vi "打开关闭文件_夹.vi"(8 "仅选中":bool, 9 "路径":path=path "C:/Users/Administrator/Desktop/技术资料/上位机/烧写软件/WR901_UpgradeTools_V3.1.3_User_20171115发布/UpgradeTools.exe", 10 "打开/关闭T":bool=TRUE, 11 "wait until completion? (T)":bool caption="等待结果后结束？(F)") -> ()   [LabVIEW 2015]
panel:
  out "standard output":string caption="标准输出"
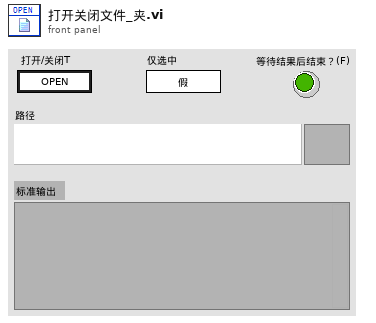
[diagram p1: front panel]
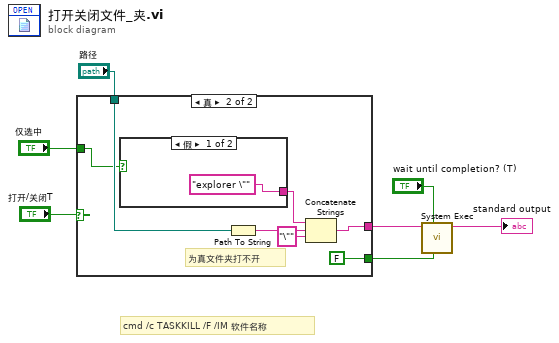
[diagram p0: block diagram]
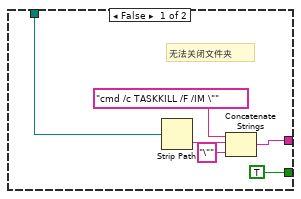
[diagram p2: hidden frame]
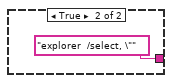
[diagram p3: hidden frame]
diagram:
  # "cmd /c TASKKILL /F /IM 软件名称"
  n1 = case shown="真" "打开/关闭T" {
    tunnel: [w12 w17] -> w7
    tunnel: "路径" -> [w11 w19]
    tunnel: [TRUE ("run minimized? (F)") FALSE ("run minimized? (F)")] -> w2
    tunnel: "仅选中" -> [_ w15]
    frame False {
      # "无法关闭文件夹"
      n2 = Strip Path(path=w11) -> (name=w10:string)  [unwired: 1 out]
      n3 = Concatenate Strings("cmd /c TASKKILL /F /IM \"" ("字符串"), w10, "\"" ("字符串")) -> (w12:string)
    }
    frame True {
      # "为真文件夹打不开"
      n4 = case shown="假" w15 {
        tunnel: ["explorer \"" ("字符串") "explorer  /select, \"" ("字符串")] -> w16
        frame False {
        }
        frame True {
        }
      }
      n5 = Path To String(path=w19) -> (string=w20:string)
      n6 = Concatenate Strings(w16, w20, "\"" ("字符串")) -> (w17:string)
    }
  }
  n7 = call <vilib>:"System Exec.vi"("run minimized? (F)"=w2, "wait until completion? (T)"="wait until completion? (T)", "command line"=w7) -> ("standard output"=→"standard output":string)  [unwired: 5 in, 3 out]
